vi "参数设置界面.vi"() -> ()   [LabVIEW 2016, in "main.lvlib"]
uses:
  main.lvlib
  control/checkbox.ctl
  DST800/DST800.lvlib
  EXO2/EXO2.lvlib
  bbe/bbe.lvlib
panel:
  in  "最小精度设置":dbl=0.01 format="%#.6f"
  in  "湖面水深设置值":u16=4
  in  "水深获取方式":bool caption="自动/手动获取湖面水深"
  in  "仪器类型":enum16{"EXO2", "BBE+NAQDO"}(ring)
  in  "DO启用":T1
  in  "BBE启用":T1 caption="启用"
  in  "BBE串口":refnum<visa-resource-name>
  in  "测试间隔":u16=4
  in  "周期运行":bool
  in  "软限位最大值":dbl=25.0 format="%#_6f m"
  in  "软限位最小值":dbl=2.0 format="%#_6f m"
  in  "单层监测时间":u32 format="%.0f s"
  in  "关闭":bool
  in  "计数器启用":T1 caption="启用"
  in  "声纳启用":T1 caption="启用"
  in  "EXO2启用":T1 caption="启用"
  in  "剖面单层深度设置":dbl format="%#_6f m"
  in  "剖面底层最小深度设定":dbl format="%#_6f m"
  in  "剖面第一层位置设定":dbl format="%#_6f m"
  in  "剖面待机位置设定":dbl format="%#_6f m"
  in  "剖面校正值设定":dbl format="%#_6f m"
  in  "编码器工程变换系数_工程值":dbl format="%#_6f m"
  in  "编码器工程变换系数_计数值":dbl format="%#_6f ps"
  in  "计数器串口":refnum<visa-resource-name>
  in  "声纳串口":refnum<visa-resource-name>
  in  "EXO2baud rate (9600)":u32=9600 caption="波特率"
  in  "EXO2串口":refnum<visa-resource-name>
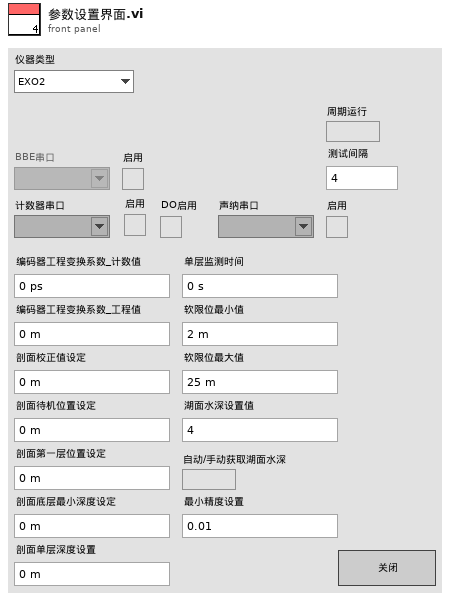
[diagram p1: front panel]
types:
  T1 = typedef "checkbox.ctl" = bool
  T2 = enum16{"open", "poll", "close", "run", "stop", "shutdown"}
  T3 = enum8{"Enabled", "Disabled", "Disabled and Grayed Out"}
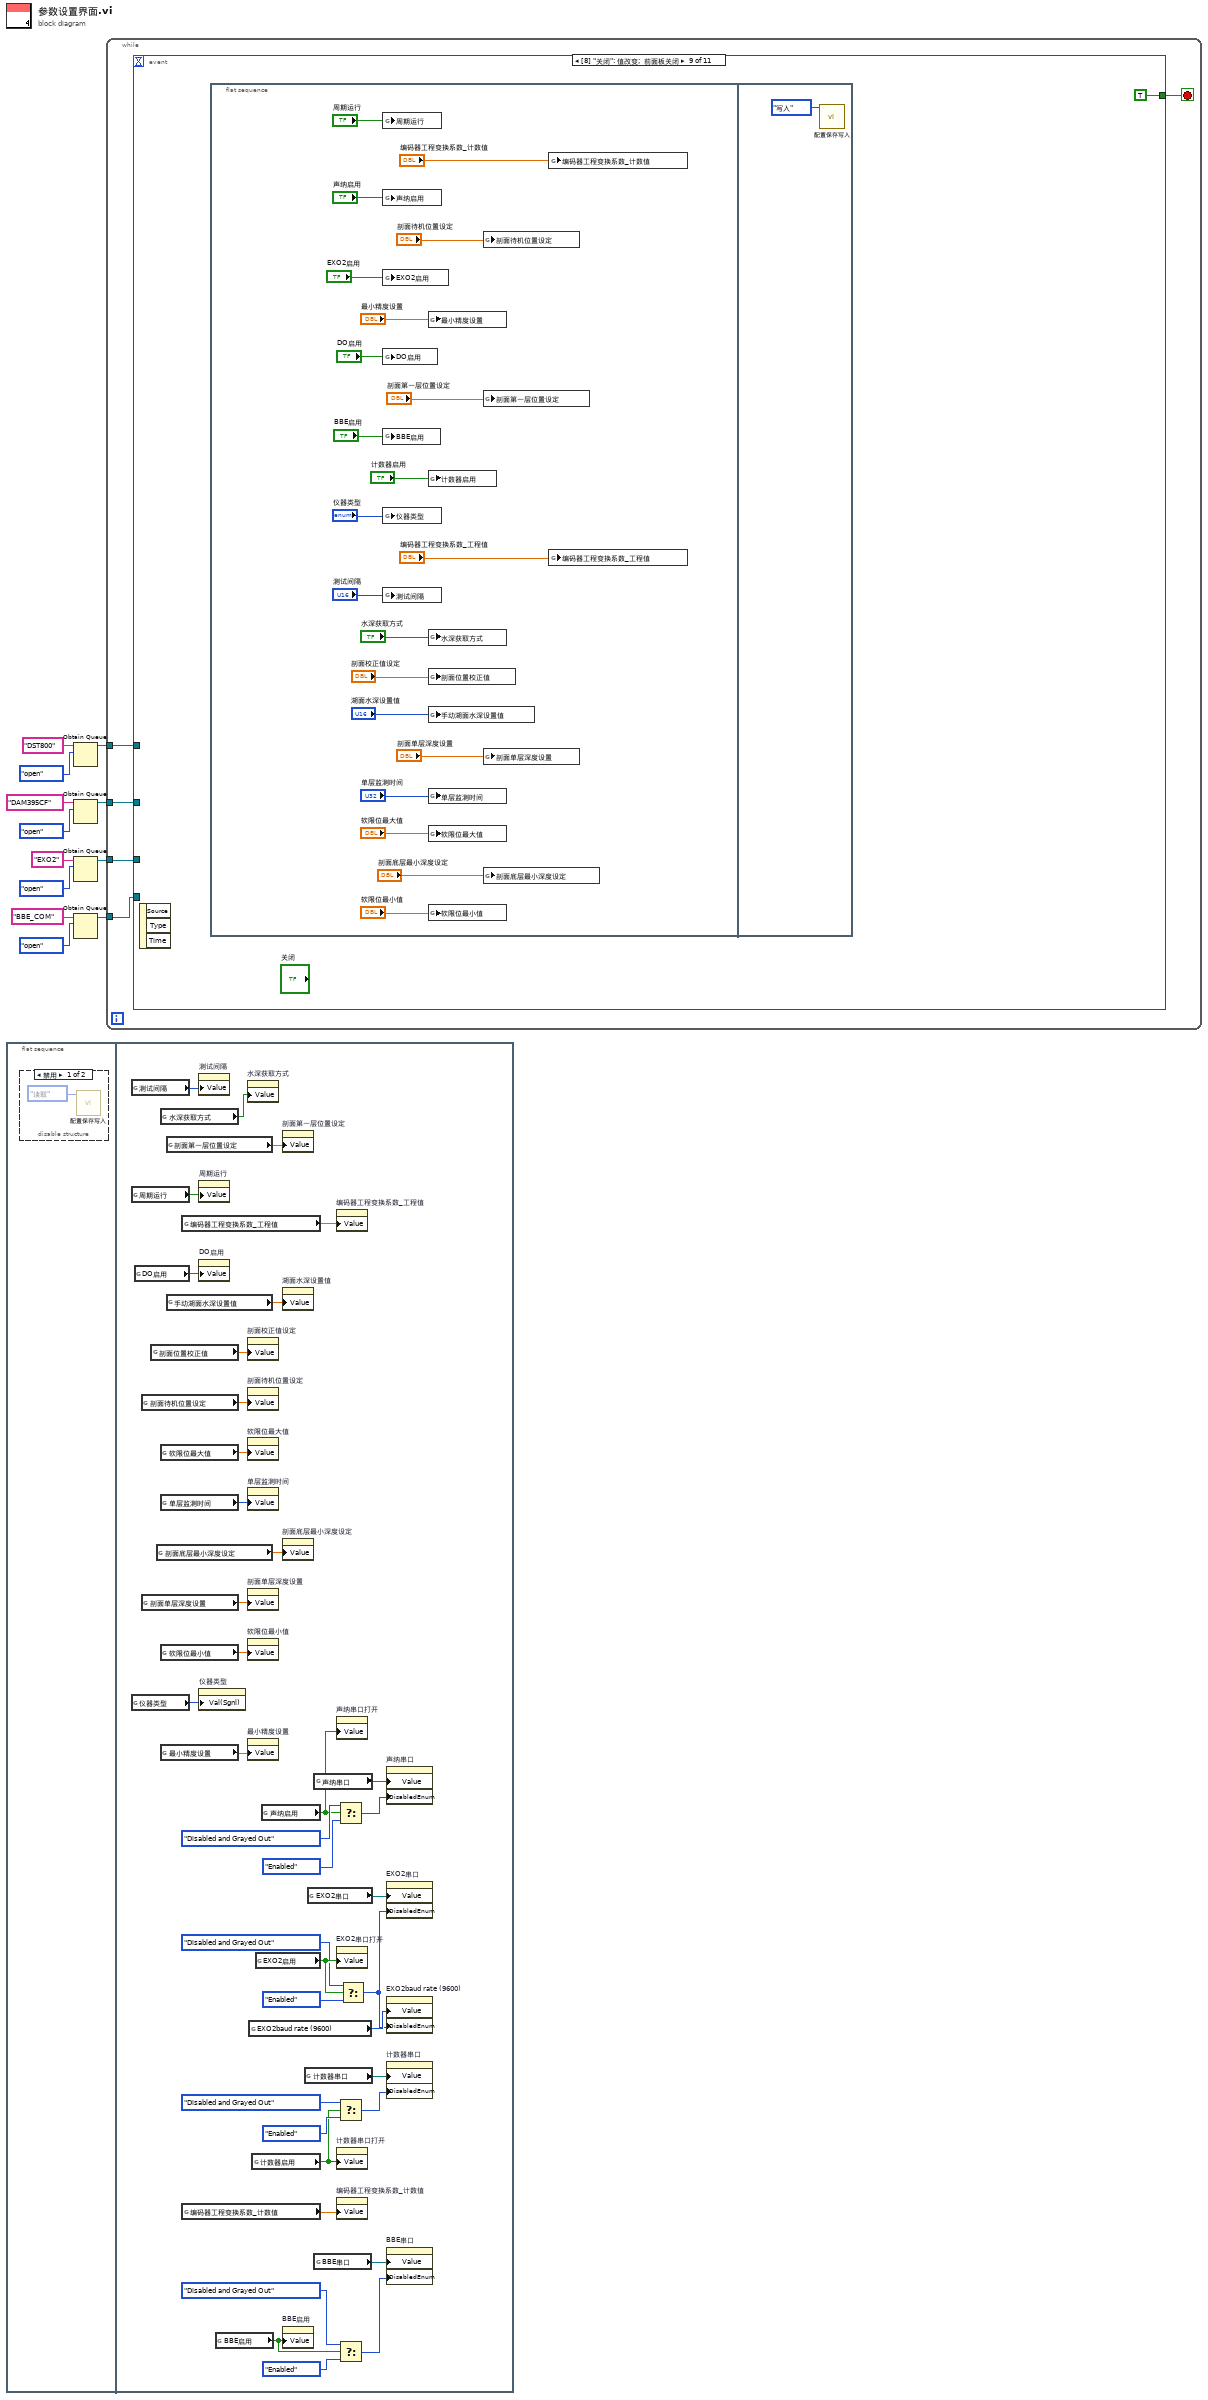
[diagram p0: block diagram]
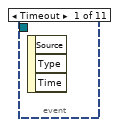
[diagram p3: hidden frame]
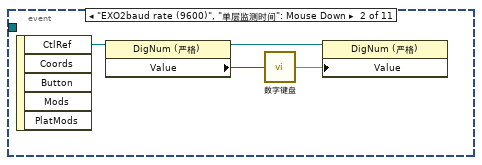
[diagram p4: hidden frame]
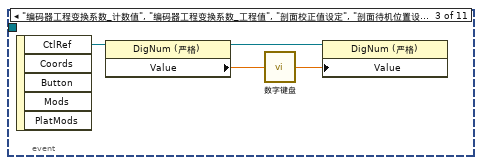
[diagram p5: hidden frame]
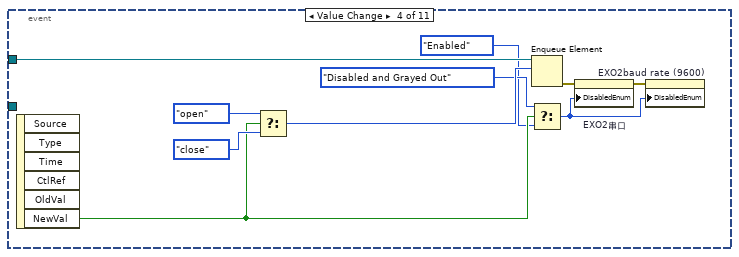
[diagram p6: hidden frame]
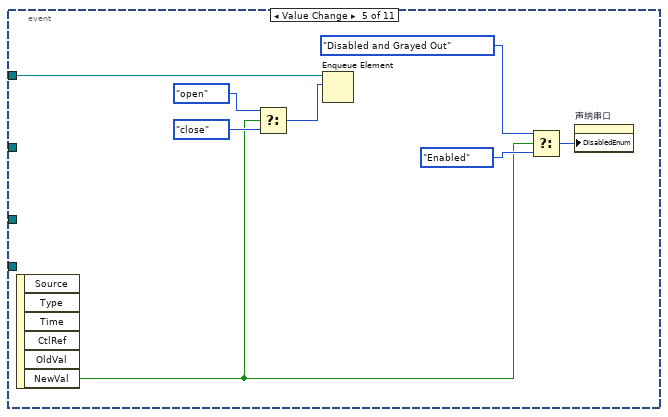
[diagram p7: hidden frame]
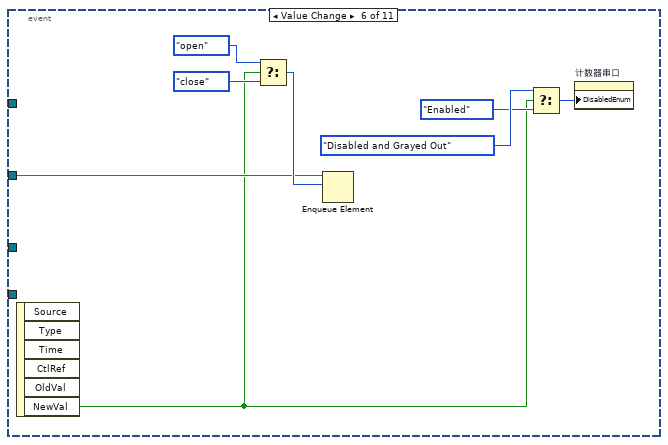
[diagram p8: hidden frame]
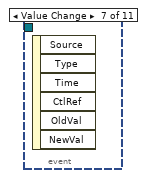
[diagram p9: hidden frame]
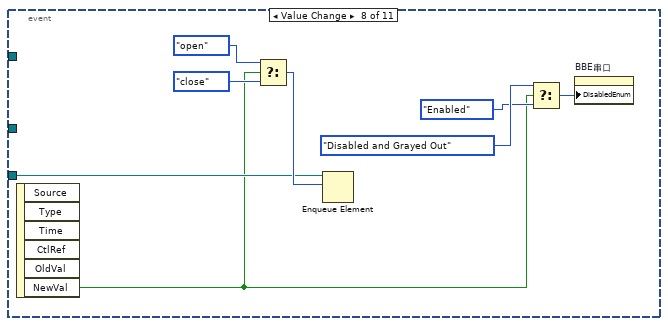
[diagram p10: hidden frame]
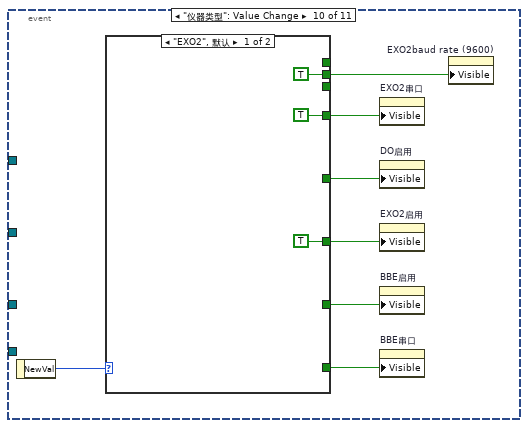
[diagram p11: hidden frame]
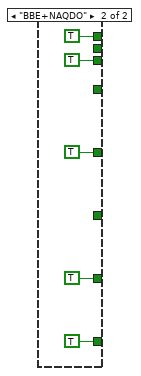
[diagram p12: hidden frame]
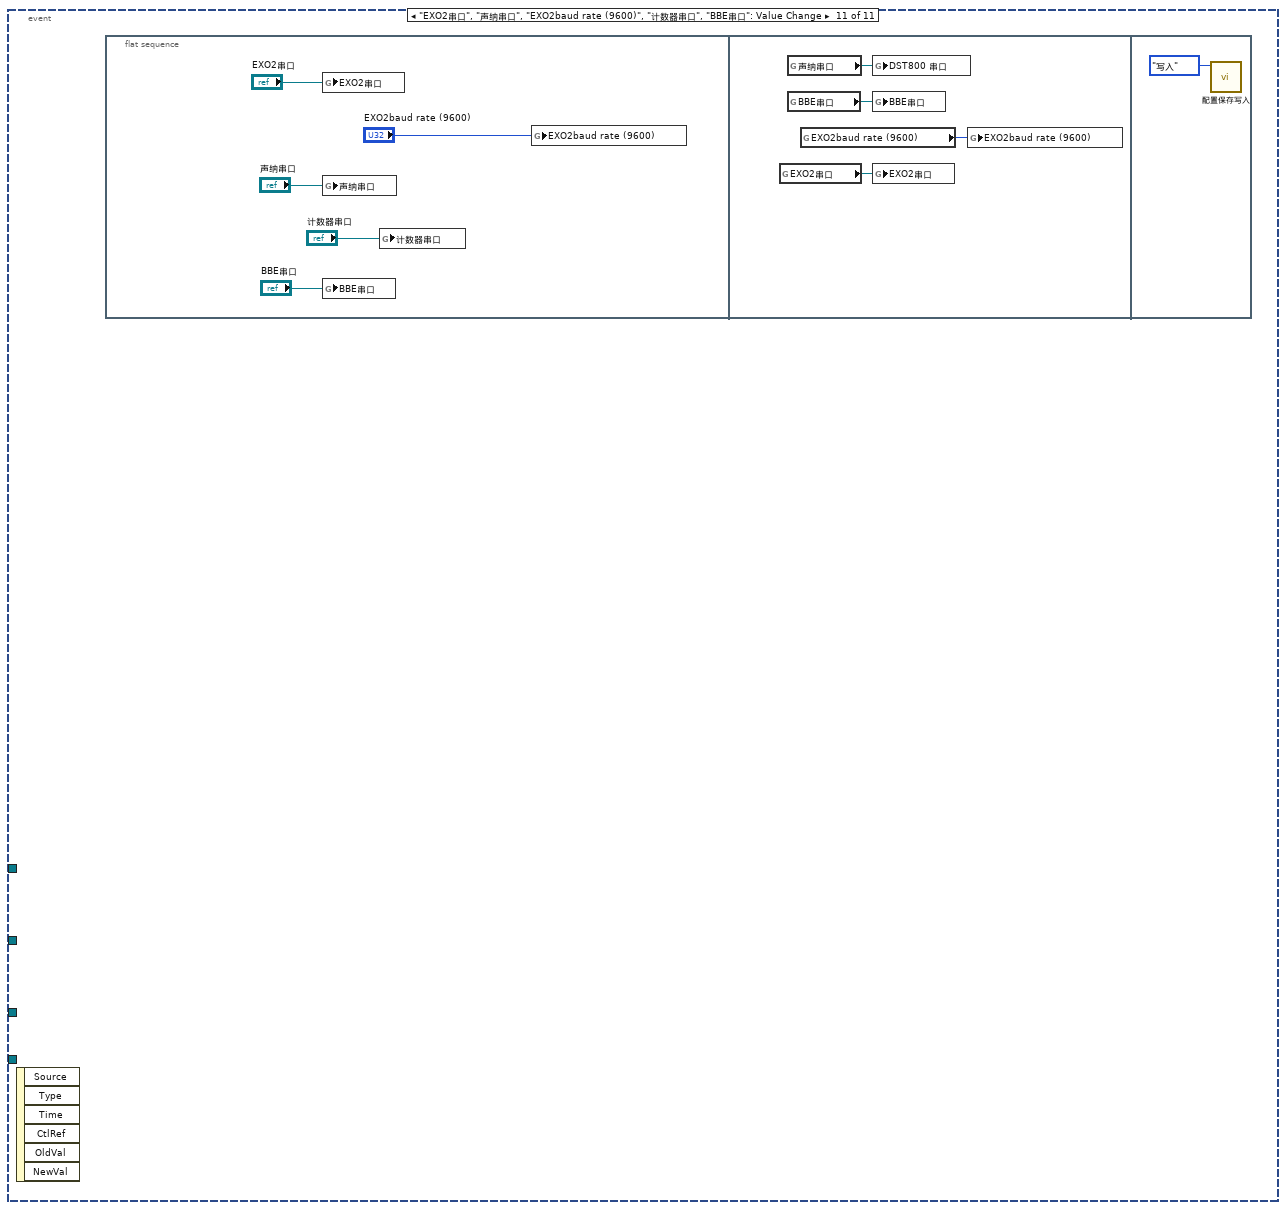
[diagram p13: hidden frame]
diagram:
  n1 = flat-sequence {
    frame #0 {
      n2 = disable-structure shown="禁用" {
        frame Disabled {
          n3 = call "配置保存写入.vi"("配置"=enum16{"读取", "写入"}."读取") -> ()  [unwired: 10 in, 1 out]
        }
        frame Enabled {
        }
      }
    }
    frame #1 {
      n4 = global read "全局断电保存变量.vi" "测试间隔"() -> (w35:u16)
      n5 = global read "全局断电保存变量.vi" "周期运行"() -> (w36:bool)
      n6 = global read "全局断电保存变量.vi" "仪器类型"() -> (w34:enum16{"EXO2", "BBE+NAQDO"})
      n7 = global read "全局断电保存变量.vi" "DO启用"() -> (w17:T1)
      n8 = global read "全局断电保存变量.vi" "剖面待机位置设定"() -> (w42:dbl)
      n9 = global read "全局断电保存变量.vi" "剖面单层深度设置"() -> (w49:dbl)
      n10 = global read "全局断电保存变量.vi" "剖面位置校正值"() -> (w46:dbl)
      n11 = global read "全局断电保存变量.vi" "剖面底层最小深度设定"() -> (w48:dbl)
      n12 = global read "全局断电保存变量.vi" "水深获取方式"() -> (w16:bool)
      n13 = global read "全局断电保存变量.vi" "软限位最大值"() -> (w38:dbl)
      n14 = global read "全局断电保存变量.vi" "单层监测时间"() -> (w40:u16)
      n15 = global read "全局断电保存变量.vi" "软限位最小值"() -> (w39:dbl)
      n16 = global read "全局断电保存变量.vi" "最小精度设置"() -> (w14:dbl)
      n17 = global read "全局断电保存变量.vi" "剖面第一层位置设定"() -> (w51:dbl)
      n18 = global read "全局断电保存变量.vi" "手动湖面水深设置值"() -> (w15:sgl)
      n19 = global read "全局断电保存变量.vi" "编码器工程变换系数_工程值"() -> (w45:dbl)
      n20 = global read "全局断电保存变量.vi" "编码器工程变换系数_计数值"() -> (w50:dbl)
      n21 = property on="测试间隔" class="DigNum (严格)"("Value"=w35) -> ()  [unwired: 2 in, 2 out]
      n22 = property on="周期运行" class="Bool (严格)"("Value"=w36) -> ()  [unwired: 2 in, 2 out]
      n23 = property on="DO启用" class="Bool (严格)"("Value"=w17) -> ()  [unwired: 2 in, 2 out]
      n24 = property on="仪器类型" class="Enum (严格)"("Val(Sgnl)"=w34) -> ()  [unwired: 2 in, 2 out]
      n25 = global read "全局断电保存变量.vi" "BBE启用"() -> (w23:T1)
      n26 = property on="水深获取方式" class="Bool (严格)"("Value"=w16) -> ()  [unwired: 2 in, 2 out]
      n27 = property on="剖面校正值设定" class="DigNum (严格)"("Value"=w46) -> ()  [unwired: 2 in, 2 out]
      n28 = property on="剖面待机位置设定" class="DigNum (严格)"("Value"=w42) -> ()  [unwired: 2 in, 2 out]
      n29 = property on="软限位最大值" class="DigNum (严格)"("Value"=w38) -> ()  [unwired: 2 in, 2 out]
      n30 = property on="单层监测时间" class="DigNum (严格)"("Value"=w40) -> ()  [unwired: 2 in, 2 out]
      n31 = property on="剖面单层深度设置" class="DigNum (严格)"("Value"=w49) -> ()  [unwired: 2 in, 2 out]
      n32 = property on="软限位最小值" class="DigNum (严格)"("Value"=w39) -> ()  [unwired: 2 in, 2 out]
      n33 = property on="最小精度设置" class="DigNum (严格)"("Value"=w14) -> ()  [unwired: 2 in, 2 out]
      n34 = global read "全局断电保存变量.vi" "EXO2baud rate (9600)"() -> (w44:u32)
      n35 = global read "全局断电保存变量.vi" "计数器启用"() -> (w27:T1)
      n36 = global read "全局断电保存变量.vi" "EXO2启用"() -> (w33:T1)
      n37 = global read "全局断电保存变量.vi" "声纳启用"() -> (w18:T1)
      n38 = property on="剖面第一层位置设定" class="DigNum (严格)"("Value"=w51) -> ()  [unwired: 2 in, 2 out]
      n39 = property on="湖面水深设置值" class="DigNum (严格)"("Value"=w15) -> ()  [unwired: 2 in, 2 out]
      n40 = property on="剖面底层最小深度设定" class="DigNum (严格)"("Value"=w48) -> ()  [unwired: 2 in, 2 out]
      n41 = property on="BBE启用" class="Bool (严格)"("Value"=w23) -> ()  [unwired: 2 in, 2 out]
      n42 = global read "全局断电保存变量.vi" "计数器串口"() -> (w47:refnum<visa-resource-name>)
      n43 = global read "全局断电保存变量.vi" "EXO2串口"() -> (w41:refnum<visa-resource-name>)
      n44 = global read "全局断电保存变量.vi" "声纳串口"() -> (w43:refnum<visa-resource-name>)
      n45 = global read "全局断电保存变量.vi" "BBE串口"() -> (w37:refnum<visa-resource-name>)
      n46 = property on="编码器工程变换系数_工程值" class="DigNum (严格)"("Value"=w45) -> ()  [unwired: 2 in, 2 out]
      n47 = property on="声纳串口打开" class="Bool (严格)"("Value"=w18) -> ()  [unwired: 2 in, 2 out]
      n48 = property on="EXO2串口打开" class="Bool (严格)"("Value"=w33) -> ()  [unwired: 2 in, 2 out]
      n49 = property on="计数器串口打开" class="Bool (严格)"("Value"=w27) -> ()  [unwired: 2 in, 2 out]
      n50 = property on="编码器工程变换系数_计数值" class="DigNum (严格)"("Value"=w50) -> ()  [unwired: 2 in, 2 out]
      n51 = Select(t=T3."Disabled and Grayed Out" ("禁用"), s=w18, f=T3."Enabled" ("禁用")) -> (s? t:f=w19:T3)
      n52 = Select(t=T3."Disabled and Grayed Out" ("禁用"), s=w27, f=T3."Enabled" ("禁用")) -> (s? t:f=w30:T3)
      n53 = Select(t=T3."Disabled and Grayed Out" ("禁用"), s=w23, f=T3."Enabled" ("禁用")) -> (s? t:f=w22:T3)
      n54 = Select(t=T3."Disabled and Grayed Out" ("禁用"), s=w33, f=T3."Enabled" ("禁用")) -> (s? t:f=w26:T3)
      n55 = property on="声纳串口" class="VISAName"("Value"=w43, "DisabledEnum"=w19) -> ()  [unwired: 2 in, 2 out]
      n56 = property on="EXO2串口" class="VISAName"("Value"=w41, "DisabledEnum"=w26) -> ()  [unwired: 2 in, 2 out]
      n57 = property on="EXO2baud rate (9600)" class="DigNum (严格)"("Value"=w44, "DisabledEnum"=w26) -> ()  [unwired: 2 in, 2 out]
      n58 = property on="计数器串口" class="VISAName"("Value"=w47, "DisabledEnum"=w30) -> ()  [unwired: 2 in, 2 out]
      n59 = property on="BBE串口" class="VISAName"("Value"=w37, "DisabledEnum"=w22) -> ()  [unwired: 2 in, 2 out]
    }
  }
  n60 = Obtain Queue(name (unnamed)="DST800" ("名称（未命名）"), element data type=enum16{"open", "poll", "close", "shutdown"}."open" ("枚举")) -> (queue out=w6:refnum<queue>)  [unwired: 3 in, 2 out]
  n61 = Obtain Queue(name (unnamed)="DAM395CF" ("名称（未命名）"), element data type=enum16{"open", "close", "poll"}."open" ("枚举")) -> (queue out=w5:refnum<queue>)  [unwired: 3 in, 2 out]
  n62 = Obtain Queue(name (unnamed)="EXO2" ("名称（未命名）"), element data type=T2."open" ("枚举")) -> (queue out=w7:refnum<queue>)  [unwired: 3 in, 2 out]
  n63 = Obtain Queue(name (unnamed)="BBE_COM" ("名称（未命名）"), element data type=enum16{"open", "close", "poll"}."open" ("枚举")) -> (queue out=w1:refnum<queue>)  [unwired: 3 in, 2 out]
  n64 = while {
    tunnel: w7 -> [w55]
    tunnel: w6 -> [w54]
    tunnel: w5 -> [w53]
    tunnel: w1 -> [w52]
    stop <- w56 stop-if-true
    n65 = event shown="[8] \"关闭\": 值改变;  前面板关闭" {
      selector: _ -> [_ _ _ _ _ _ _ _ _ _ _]
      dyn-events: _ -> [_ _ _ _ _ _ _ _ _ _ _]
      timeout: _ -> [_ _ _ _ _ _ _ _ _ _ _]
      tunnel: [_ _ _ _ _ _ _ _ TRUE _ _] -> w56
      tunnel: w55 -> [_ _ _ w74 _ _ _ _ _ _ _]
      tunnel: w54 -> [_ _ _ _ w81 _ _ _ _ _ _]
      tunnel: w53 -> [_ _ _ _ _ w89 _ _ _ _ _]
      tunnel: w52 -> [_ _ _ _ _ _ _ w97 _ _ _]
      event Timeout {
        n66 = event-data() -> ()  [unwired: 1 in, 3 out]
      }
      event "EXO2baud rate (9600)", "单层监测时间": Mouse Down {
        n67 = event-data() -> ("CtlRef"=w60:refnum<vi>)  [unwired: 1 in, 4 out]
        n68 = property class="DigNum (严格)"(reference=w60) -> (reference out=w57:refnum<vi>, "Value"=w59:u32)  [unwired: 1 in, 1 out]
        n69 = call "数字键盘.vi"("OldNumber"=w59) -> ("NewNumber"=w58:dbl)
        n70 = property class="DigNum (严格)"(reference=w57, "Value"=w58) -> ()  [unwired: 1 in, 2 out]
      }
      event "编码器工程变换系数_计数值", "编码器工程变换系数_工程值", "剖面校正值设定", "剖面待机位置设定", "剖面第一层位置设定", "剖面底层最小深度设定", "剖面单层深度设置", "软限位最小值", "软限位最大值": Mouse Down {
        n71 = event-data() -> ("CtlRef"=w64:refnum<vi>)  [unwired: 1 in, 4 out]
        n72 = property class="DigNum (严格)"(reference=w64) -> (reference out=w61:refnum<vi>, "Value"=w63:dbl)  [unwired: 1 in, 1 out]
        n73 = call "数字键盘.vi"("OldNumber"=w63) -> ("NewNumber"=w62:dbl)
        n74 = property class="DigNum (严格)"(reference=w61, "Value"=w62) -> ()  [unwired: 1 in, 2 out]
      }
      event Value Change {
        n75 = event-data() -> ("NewVal"=w70:T1)  [unwired: 1 in, 5 out]
        n76 = Select(t=T2."open" ("枚举"), s=w70, f=T2."close" ("枚举")) -> (s? t:f=w71:T2)
        n77 = Enqueue Element(queue=w74, element=w71) -> (error out=w65:errorcluster)  [unwired: 2 in, 2 out]
        n78 = Select(t=T3."Disabled and Grayed Out" ("禁用"), s=w70, f=T3."Enabled" ("禁用")) -> (s? t:f=w67:T3)
        n79 = property on="EXO2串口" class="VISAName"(error in=w65, "DisabledEnum"=w67) -> (error out=w66:errorcluster)  [unwired: 1 in, 1 out]
        n80 = property on="EXO2baud rate (9600)" class="DigNum (严格)"(error in=w66, "DisabledEnum"=w67) -> ()  [unwired: 1 in, 2 out]
      }
      event Value Change {
        n81 = event-data() -> ("NewVal"=w76:T1)  [unwired: 1 in, 5 out]
        n82 = Select(t=enum16{"open", "poll", "close", "shutdown"}."open" ("枚举"), s=w76, f=enum16{"open", "poll", "close", "shutdown"}."close" ("枚举")) -> (s? t:f=w82:enum16{"open", "poll", "close", "shutdown"})
        n83 = Enqueue Element(queue=w81, element=w82) -> ()  [unwired: 2 in, 3 out]
        n84 = Select(t=T3."Disabled and Grayed Out" ("禁用"), s=w76, f=T3."Enabled" ("禁用")) -> (s? t:f=w75:T3)
        n85 = property on="声纳串口" class="VISAName"("DisabledEnum"=w75) -> ()  [unwired: 2 in, 2 out]
      }
      event Value Change {
        n86 = event-data() -> ("NewVal"=w84:T1)  [unwired: 1 in, 5 out]
        n87 = Select(t=enum16{"open", "close", "poll"}."open" ("枚举"), s=w84, f=enum16{"open", "close", "poll"}."close" ("枚举")) -> (s? t:f=w90:enum16{"open", "close", "poll"})
        n88 = Enqueue Element(queue=w89, element=w90) -> ()  [unwired: 2 in, 3 out]
        n89 = Select(t=T3."Disabled and Grayed Out" ("禁用"), s=w84, f=T3."Enabled" ("禁用")) -> (s? t:f=w83:T3)
        n90 = property on="计数器串口" class="VISAName"("DisabledEnum"=w83) -> ()  [unwired: 2 in, 2 out]
      }
      event Value Change {
        n91 = event-data() -> ()  [unwired: 1 in, 6 out]
      }
      event Value Change {
        n92 = event-data() -> ("NewVal"=w91:T1)  [unwired: 1 in, 5 out]
        n93 = Select(t=enum16{"open", "close", "poll"}."open" ("枚举"), s=w91, f=enum16{"open", "close", "poll"}."close" ("枚举")) -> (s? t:f=w98:enum16{"open", "close", "poll"})
        n94 = Enqueue Element(queue=w97, element=w98) -> ()  [unwired: 2 in, 3 out]
        n95 = Select(t=T3."Disabled and Grayed Out" ("禁用"), s=w91, f=T3."Enabled" ("禁用")) -> (s? t:f=w92:T3)
        n96 = property on="BBE串口" class="VISAName"("DisabledEnum"=w92) -> ()  [unwired: 2 in, 2 out]
      }
      event "关闭": Value Change; Panel Close {
        n97 = event-data() -> ()  [unwired: 1 in, 3 out]
        n98 = flat-sequence {
          frame #0 {
            n99 = global write "全局断电保存变量.vi" "周期运行"("周期运行") -> ()
            n100 = global write "全局断电保存变量.vi" "声纳启用"("声纳启用") -> ()
            n101 = global write "全局断电保存变量.vi" "EXO2启用"("EXO2启用") -> ()
            n102 = global write "全局断电保存变量.vi" "DO启用"("DO启用") -> ()
            n103 = global write "全局断电保存变量.vi" "BBE启用"("BBE启用") -> ()
            n104 = global write "全局断电保存变量.vi" "仪器类型"("仪器类型") -> ()
            n105 = global write "全局断电保存变量.vi" "测试间隔"("测试间隔") -> ()
            n106 = global write "全局断电保存变量.vi" "最小精度设置"("最小精度设置") -> ()
            n107 = global write "全局断电保存变量.vi" "计数器启用"("计数器启用") -> ()
            n108 = global write "全局断电保存变量.vi" "水深获取方式"("水深获取方式") -> ()
            n109 = global write "全局断电保存变量.vi" "剖面位置校正值"("剖面校正值设定") -> ()
            n110 = global write "全局断电保存变量.vi" "手动湖面水深设置值"("湖面水深设置值") -> ()
            n111 = global write "全局断电保存变量.vi" "单层监测时间"("单层监测时间") -> ()
            n112 = global write "全局断电保存变量.vi" "软限位最大值"("软限位最大值") -> ()
            n113 = global write "全局断电保存变量.vi" "软限位最小值"("软限位最小值") -> ()
            n114 = global write "全局断电保存变量.vi" "剖面待机位置设定"("剖面待机位置设定") -> ()
            n115 = global write "全局断电保存变量.vi" "剖面第一层位置设定"("剖面第一层位置设定") -> ()
            n116 = global write "全局断电保存变量.vi" "剖面单层深度设置"("剖面单层深度设置") -> ()
            n117 = global write "全局断电保存变量.vi" "剖面底层最小深度设定"("剖面底层最小深度设定") -> ()
            n118 = global write "全局断电保存变量.vi" "编码器工程变换系数_计数值"("编码器工程变换系数_计数值") -> ()
            n119 = global write "全局断电保存变量.vi" "编码器工程变换系数_工程值"("编码器工程变换系数_工程值") -> ()
          }
          frame #1 {
            n120 = call "配置保存写入.vi"("配置"=enum16{"读取", "写入"}."写入") -> ()  [unwired: 10 in, 1 out]
          }
        }
      }
      event "仪器类型": Value Change {
        n121 = event-data() -> ("NewVal"=w128:enum16{"EXO2", "BBE+NAQDO"})  [unwired: 1 in]
        n122 = case shown="\"EXO2\", 默认" w128 {
          tunnel: [TRUE ("可见") _] -> w127
          tunnel: [TRUE ("可见") _] -> w126
          tunnel: [TRUE ("可见") _] -> w125
          tunnel: [_ TRUE] -> w124
          tunnel: [_ TRUE] -> w123
          tunnel: [_ TRUE] -> w122
          tunnel: [_ TRUE] -> _
          tunnel: [_ T1 TRUE ("值(信号)")] -> _
          frame "EXO2", Default {
          }
          frame "BBE+NAQDO" {
          }
        }
        n123 = property on="EXO2串口" class="VISAName"("Visible"=w126) -> ()  [unwired: 2 in, 2 out]
        n124 = property on="DO启用" class="Bool (严格)"("Visible"=w122) -> ()  [unwired: 2 in, 2 out]
        n125 = property on="EXO2启用" class="Bool (严格)"("Visible"=w127) -> ()  [unwired: 2 in, 2 out]
        n126 = property on="BBE启用" class="Bool (严格)"("Visible"=w123) -> ()  [unwired: 2 in, 2 out]
        n127 = property on="BBE串口" class="VISAName"("Visible"=w124) -> ()  [unwired: 2 in, 2 out]
        n128 = property on="EXO2baud rate (9600)" class="DigNum (严格)"("Visible"=w125) -> ()  [unwired: 2 in, 2 out]
      }
      event "EXO2串口", "声纳串口", "EXO2baud rate (9600)", "计数器串口", "BBE串口": Value Change {
        n129 = event-data() -> ()  [unwired: 1 in, 6 out]
        n130 = flat-sequence {
          frame #0 {
            n131 = global write "全局断电保存变量.vi" "EXO2串口"("EXO2串口") -> ()
            n132 = global write "全局断电保存变量.vi" "声纳串口"("声纳串口") -> ()
            n133 = global write "全局断电保存变量.vi" "BBE串口"("BBE串口") -> ()
            n134 = global write "全局断电保存变量.vi" "计数器串口"("计数器串口") -> ()
            n135 = global write "全局断电保存变量.vi" "EXO2baud rate (9600)"("EXO2baud rate (9600)") -> ()
          }
          frame #1 {
            n136 = global read "全局断电保存变量.vi" "EXO2串口"() -> (w144:refnum<visa-resource-name>)
            n137 = global read "全局断电保存变量.vi" "声纳串口"() -> (w142:refnum<visa-resource-name>)
            n138 = global read "全局断电保存变量.vi" "BBE串口"() -> (w145:refnum<visa-resource-name>)
            n139 = global read "全局断电保存变量.vi" "EXO2baud rate (9600)"() -> (w143:u32)
            n140 = global write "DST800全局变量.vi" "DST800 串口"(w142) -> ()
            n141 = global write "过程变量.vi" "BBE串口"(w145) -> ()
            n142 = global write "EXO2全局变量.vi" "EXO2串口"(w144) -> ()
            n143 = global write "EXO2全局变量.vi" "EXO2baud rate (9600)"(w143) -> ()
          }
          frame #2 {
            n144 = call "配置保存写入.vi"("配置"=enum16{"读取", "写入"}."写入") -> ()  [unwired: 10 in, 1 out]
          }
        }
      }
    }
  }
